vi "FTW-Panel-FrontPanel-Close.vi"(8 "error in":errorcluster, 11 "VI Ref":refnum<vi>) -> (0 "error out":errorcluster, 3 "VI Ref out":refnum<vi>)   [LabVIEW 2013]
panel:
  # "Inputs"
  # "Outputs"
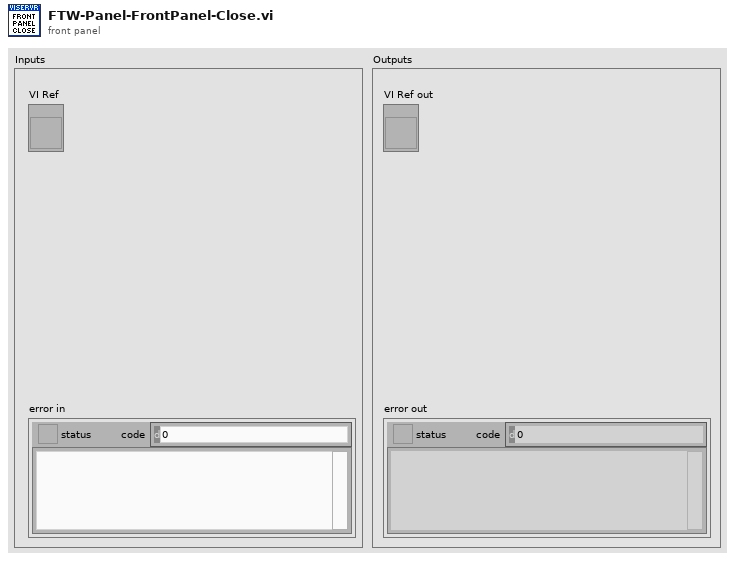
[diagram p1: front panel]
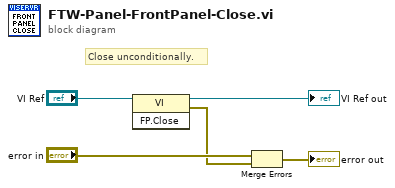
[diagram p0: block diagram]
diagram:
  # "Close unconditionally."
  n1 = invoke class="VI" method="FP.Close"(reference="VI Ref") -> (reference out=→"VI Ref out":refnum<vi>, error out=w2:errorcluster)  [unwired: 2 in, 1 out]
  n2 = Merge Errors("error in", w2) -> (→"error out":errorcluster)
